vi "Save Panel Image to File.vi"(4 "Position":cluster{"Left":u32, "Top":u32}, 5 "Image Format":enum16{"JPEG", "PNG", "BMP"}(ring), 6 "Picture Dimensions":cluster{"Width":u32, "Height":u32}, 7 "Bit Depth":enum16{"1-bit", "4-bit", "8-bit", "24-bit"}(ring)=enum."24-bit", 8 "error in (no error)":errorcluster, 10 "VI Name\n(empty - caller VI)":string, 11 "Path (empty - prompt)":path) -> (0 "error out":errorcluster, 3 "Image Path":path)   [LabVIEW 2011]
doc: "This VI will take the contents of a picture control / indicator and save it to file as either a JPEG, BMP, or PNG file. Run this VI in as a subVI of the main VI where the picture control / indicator is located. \n\nRequirements for using this VI are that the picture control MUST be entirely visible on the screen and it MUST NOT have a label showing. To make sure that this is the case, go to the control, right-click, choose show->label and verify that the label is not showing. \n\nThe VI obtains the picture image, prompts the user for a location to save the file, and then saves the image to disk.\n\nNOTE: This VI DOES NOT take the picture as inputs, only information about the picture's dimesions and location on the screen. Do not think that the picture must be wired to the VI.\n\nThis VI takes 6 inputs:\n\nVI Path: This is the path of the VI where the picture control is.\n\nImage Fomat: The format of the image file (JPEG, BMP, or PNG)\n\nBit Depth: Image depth of the file (1-bit, 4-bit, 8-bit, 24-bit)\n\nPicture Dimensions: Size of the picture in pixels. (get this from the Draw Area Size attribute)\n\nPosition: Location of the picture control on the front panel. (get from the Position attribute)\n\nError In: Error In cluster.\n\nThe VI returns 2 outputs:\n\nImage Path: The path of the image file where the picture was saved.\n\nError out: Error out cluster."
panel:
  # "Run this VI as a subVI and pass it the appropriate information."
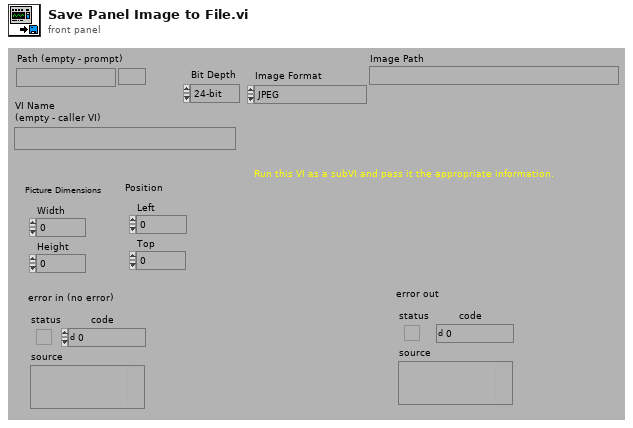
[diagram p1: front panel]
types:
  T1 = cluster{"left":i16, "top":i16, "right":i16, "bottom":i16}
  T2 = typedef "imagedata.ctl" = cluster{"image type":i32, "image depth":i32, "image":u8[], "mask":u8[], "colors":u32[], "Rectangle":cluster{"left":i16, "top":i16, "right":i16, "bottom":i16}}
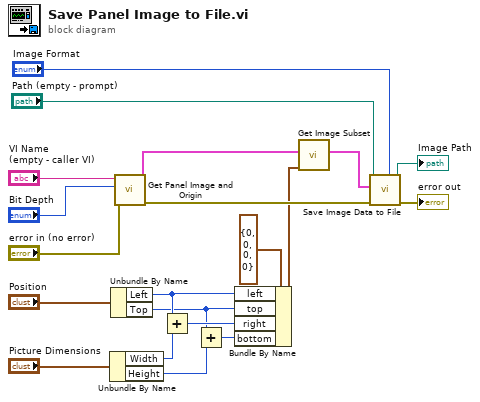
[diagram p0: block diagram]
diagram:
  n1 = Unbundle By Name("Picture Dimensions") -> ("Width"=w5:u32, "Height"=w3:u32)
  n2 = Unbundle By Name("Position") -> ("Left"=w6:u32, "Top"=w1:u32)
  n3 = call "Get Panel Image and Origin.vi"("error in (no error)"="error in (no error)", "Bit Depth"="Bit Depth", "vi name"="VI Name\n(empty - caller VI)") -> ("error out"=w18:errorcluster, "image data"=w12:T2)  [unwired: 7 out]
  n4 = Add(x=w6, y=w5) -> (x+y=w4:u32)
  n5 = Add(x=w1, y=w3) -> (x+y=w2:u32)
  n6 = Bundle By Name(cluster=T1 {"left"=0, "top"=0, "right"=0, "bottom"=0} ("subset rect"), "left"=w6, "top"=w1, "right"=w4, "bottom"=w2) -> (w9:T1)
  n7 = call <vilib>:"Get Image Subset.vi"("subset rect"=w9, "image data"=w12) -> ("image subset"=w11:T2)  [unwired: 5 out]
  n8 = call "Save Image Data to File.vi"("Image Format"="Image Format", "error in (no error)"=w18, "image data"=w11, "Path"="Path (empty - prompt)") -> ("error out"=→"error out":errorcluster, "Path Out"=→"Image Path":path)  [unwired: 2 in, 4 out]
